vi "3D_Contour_Plot_Merge_VI.vi"() -> ()   [LabVIEW 2020]
uses:
  <vilib>/Math Plots/3D Math Plots/3D Contour/3D Contour XCtrl/3D Contour.xctl
  <vilib>/Math Plots/3D Math Plots/3D Contour/3D Contour Datatype/Public/Plot Helper (Matrix).vi
  <vilib>/Math Plots/3D Math Plots/3D Contour/3D Contour Datatype/3D Contour Datatype.lvclass
panel:
  out "3D Contour":refnum<class "3D Plot Datatype.lvclass">[](xcontrol)
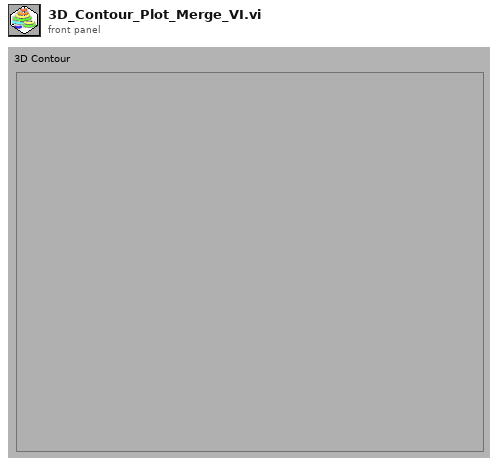
[diagram p1: front panel]
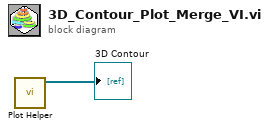
[diagram p0: block diagram]
diagram:
  n1 = call-poly <vilib>:"Plot Helper.vi"() -> ("3D Plot lvclass Array out"=→"3D Contour":refnum<class "3D Plot Datatype.lvclass">[])  [unwired: 6 in, 5 out]
